vi "Shoot_ReadDash.vi"   [LabVIEW 2025]
uses:
  <vilib>/Rock Robotics/Network Tables/NT Read Number.vi
  Shoot_Global.vi
  <vilib>/Rock Robotics/Network Tables/NT Read Boolean.vi
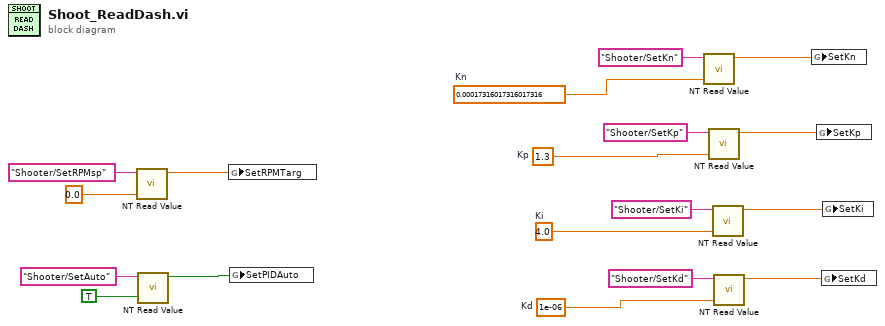
[diagram p0: block diagram]
diagram:
  w3 = 1.3  # Kp
  w2 = 4.0  # Ki
  w1 = 1e-06  # Kd
  w4 = 0.00017316017316017316  # Kn
  n1 = call-poly <vilib>:"NT Read Value.vi"("default value"=0.0, "name"="Shooter/SetRPMsp") -> ("value"=w18:dbl)  [unwired: 7 in, 2 out]
  n2 = call-poly <vilib>:"NT Read Value.vi"("default value"=TRUE, "name"="Shooter/SetAuto") -> ("value"=w15:bool)  [unwired: 7 in, 2 out]
  n3 = global write "Shoot_Global.vi" "SetRPMTarg"(w18) -> ()
  n4 = global write "Shoot_Global.vi" "SetPIDAuto"(w15) -> ()
  n5 = call-poly <vilib>:"NT Read Value.vi"("default value"=w4, "name"="Shooter/SetKn") -> ("value"=w12:dbl)  [unwired: 7 in, 2 out]
  n6 = call-poly <vilib>:"NT Read Value.vi"("default value"=w3, "name"="Shooter/SetKp") -> ("value"=w10:dbl)  [unwired: 7 in, 2 out]
  n7 = call-poly <vilib>:"NT Read Value.vi"("default value"=w2, "name"="Shooter/SetKi") -> ("value"=w8:dbl)  [unwired: 7 in, 2 out]
  n8 = call-poly <vilib>:"NT Read Value.vi"("default value"=w1, "name"="Shooter/SetKd") -> ("value"=w6:dbl)  [unwired: 7 in, 2 out]
  n9 = global write "Shoot_Global.vi" "SetKn"(w12) -> ()
  n10 = global write "Shoot_Global.vi" "SetKp"(w10) -> ()
  n11 = global write "Shoot_Global.vi" "SetKd"(w6) -> ()
  n12 = global write "Shoot_Global.vi" "SetKi"(w8) -> ()
